vi "Set.vi"(7 "ICAN":refnum<class "ICAN.lvclass">, 8 "Error In":errorcluster, 9 "Node-ID":u8, 10 "SDO Manager":refnum<class "SDO Manager.lvclass">, 11 "reference in":refnum<class "Heartbeat.lvclass">) -> (0 "Error Out":errorcluster, 1 "Timed Outs?":bool[](array[boolean]), 2 "Node-IDs":u8[](array[numeric]), 3 "reference out":refnum<class "Heartbeat.lvclass">)   [LabVIEW 2024, in "CANopen Master.lvlib" / "Heartbeat.lvclass"]
uses:
  Heartbeat.lvclass
  SDO Manager/SDO Manager.lvclass
  HAL/HAL/Protocols/ICAN/ICAN.lvclass
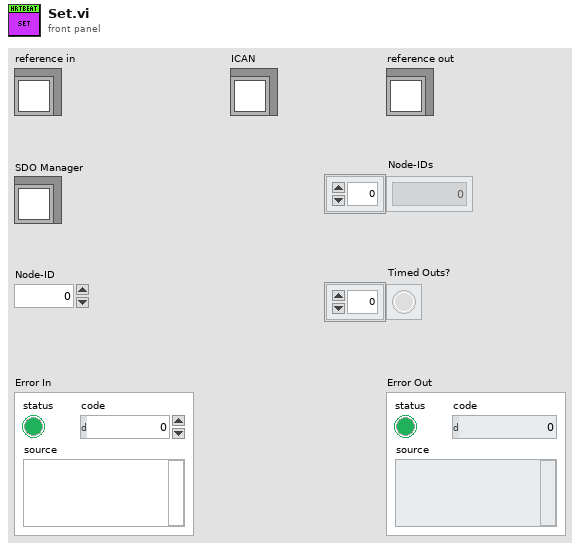
[diagram p1: front panel]
types:
  T1 = typedef "CANopen Master.lvlib/Heartbeat.lvclass/ObjectAttributes.ctl" = cluster{"Heartbeats":map{u8, cluster{"Period":u16, "Timeout":u16, "Last Beat":refnum<class "Time Stamp.lvclass">}}}
  T2 = map{u8, cluster{"Period":u16, "Timeout":u16, "Last Beat":refnum<class "Time Stamp.lvclass">}}
  T3 = cluster{"Period":u16, "Timeout":u16, "Last Beat":refnum<class "Time Stamp.lvclass">}
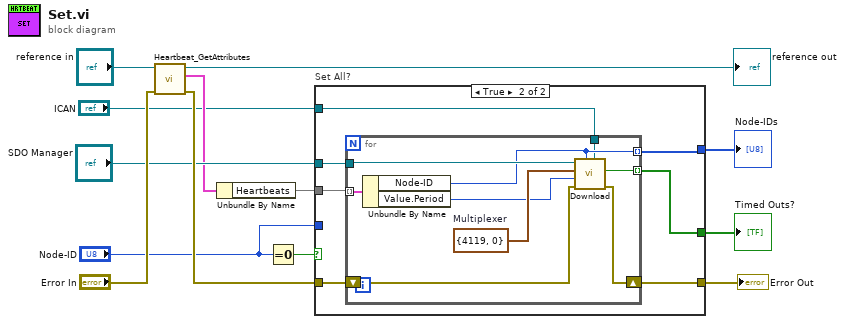
[diagram p0: block diagram]
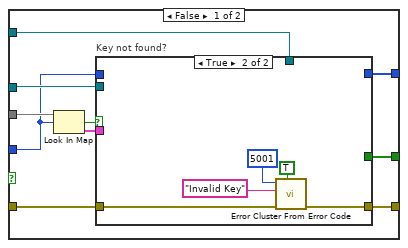
[diagram p2: hidden frame]
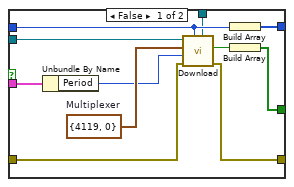
[diagram p3: hidden frame]
diagram:
  n1 = call "Heartbeat_GetAttributes.vi"("Error In"="Error In", "reference in"="reference in") -> ("Error Out"=w9:errorcluster, "Data"=w6:T1, "reference out"=→"reference out":refnum<class "Heartbeat.lvclass">)  [unwired: 6 in, 1 out]
  n2 = Unbundle By Name(w6) -> ("Heartbeats"=w5:T2)
  n3 = Equal To 0?(x="Node-ID") -> (x = 0?=w10:bool)
  n4 = case "Set All?" shown="True" w10 {
    tunnel: w9 -> [w21 w46]
    tunnel: [w20 w45] -> w8
    tunnel: "SDO Manager" -> [w22 w44]
    tunnel: [w19 w43] -> w3
    tunnel: w5 -> [w23 w42]
    tunnel: "Node-ID" -> [w17 _]
    tunnel: [w15 w41] -> w2
    tunnel: "ICAN" -> [w14 w40]
    frame False {
      n5 = Look In Map(map=w23, key=w17) -> (key not found?=w16:bool, value=w18:T3)  [unwired: 1 in]
      n6 = case "Key not found?" shown="True" w16 {
        tunnel: w22 -> [w32 _]
        tunnel: w21 -> [w31 w39]
        tunnel: [w30 w38] -> w20
        tunnel: [w28 _] -> w19
        tunnel: w18 -> [w29 _]
        tunnel: w17 -> [w26 _]
        tunnel: [w25 _] -> w15
        tunnel: w14 -> [w24 _]
        frame False {
          w34 = cluster{"Index":u16, "Sub-Index":u8} {"Index"=4119, "Sub-Index"=0}  # Multiplexer
          n7 = Unbundle By Name(w29) -> ("Period"=w33:u16)
          n8 = call "Download.vi"("ICAN"=w24, "Node-ID"=w26, "error in"=w31, "Value"=w33, "Multiplexer"=w34, "SDO Manager in"=w32) -> ("error out"=w30:errorcluster, "Success?"=w27:bool)  [unwired: 3 in, 1 out]
          n9 = Build Array(w26) -> (w25:u8[])
          n10 = Build Array(w27) -> (w28:bool[])
        }
        frame True {
          n11 = call <vilib>:"Error Cluster From Error Code.vi"("show call chain? (False)"=TRUE, "error in (no error)"=w39, "error message (\"\")"="Invalid Key" ("error message (\"\")"), "error code (0)"=5001) -> ("error out"=w38:errorcluster)  [unwired: 5 in]
        }
      }
    }
    frame True {
      n12 = for {
        tunnel: w42 -> [w55] mode=indexing
        shift-right: [w51] -> w45
        shift-left: w46 -> [w52]
        tunnel: w44 -> [w54]
        tunnel: [w49] -> w43 mode=indexing
        tunnel: [w48] -> w41 mode=indexing
        tunnel: w40 -> [w47]
        w53 = cluster{"Index":u16, "Sub-Index":u8} {"Index"=4119, "Sub-Index"=0}  # Multiplexer
        n13 = Unbundle By Name(w55) -> ("Node-ID"=w48:u8, "Value.Period"=w50:u16)
        n14 = call "Download.vi"("ICAN"=w47, "Node-ID"=w48, "error in"=w52, "Value"=w50, "Multiplexer"=w53, "SDO Manager in"=w54) -> ("error out"=w51:errorcluster, "Success?"=w49:bool)  [unwired: 3 in, 1 out]
      }
    }
  }
  "Error Out" <- w8
  "Timed Outs?" <- w3
  "Node-IDs" <- w2
